vi "比率.vi"(10 "Fail 个数":dbl, 11 "Pass 个数":dbl) -> (1 "result":T1, 2 "fail 率":dbl, 3 "pass率":dbl)   [LabVIEW 2017]
panel:
  out "x/y 2":dbl
  out "x*y":dbl
  out "x/y":dbl
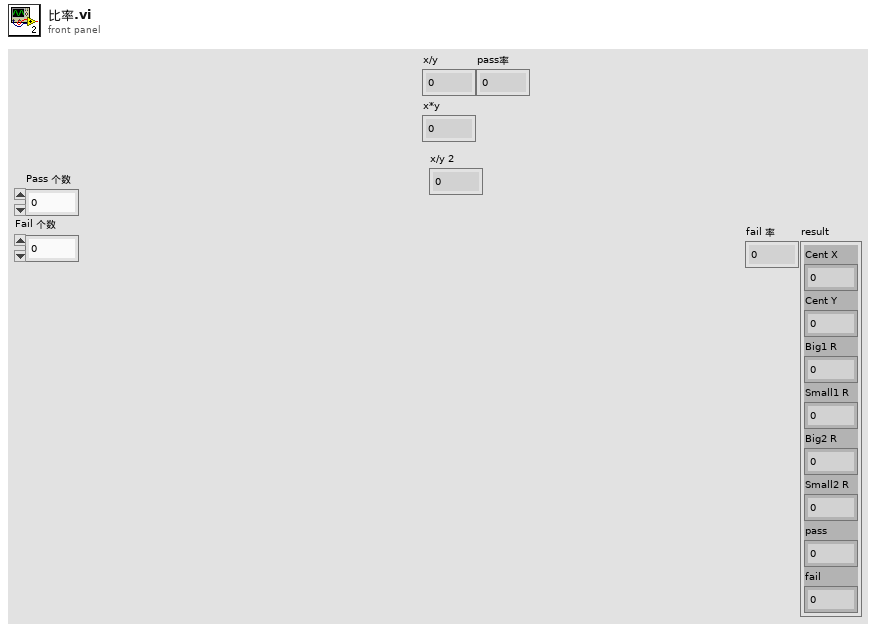
[diagram p1: front panel]
types:
  T1 = cluster{"Cent X":dbl, "Cent Y":dbl, "Big1 R":dbl, "Small1 R":dbl, "Big2 R":dbl, "Small2 R":dbl, "pass":dbl, "fail":dbl}
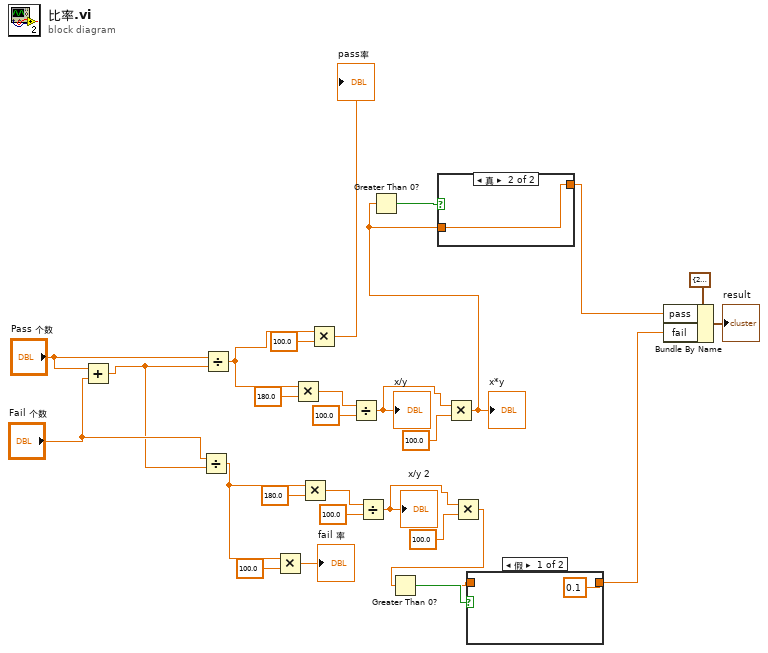
[diagram p0: block diagram]
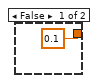
[diagram p3: hidden frame]
diagram:
  n1 = Add(x="Pass 个数", y="Fail 个数") -> (x+y=w19:dbl)
  n2 = Divide(x="Fail 个数", y=w19) -> (x/y=w10:dbl)
  n3 = Divide(x="Pass 个数", y=w19) -> (x/y=w13:dbl)
  n4 = Multiply(x=w10, y=100.0) -> (x*y=→"fail 率":dbl)
  n5 = Multiply(x=w13, y=180.0) -> (x*y=w23:dbl)
  n6 = Multiply(x=w10, y=180.0) -> (x*y=w16:dbl)
  n7 = Multiply(x=w13, y=100.0) -> (x*y=→"pass率":dbl)
  n8 = Divide(x=w23, y=100.0) -> (x/y=w22:dbl)
  "x/y" <- w22
  n9 = Divide(x=w16, y=100.0) -> (x/y=w17:dbl)
  "x/y 2" <- w17
  n10 = Multiply(x=w22, y=100.0) -> (x*y=w3:dbl)
  "x*y" <- w3
  n11 = Greater Than 0?(x=w3) -> (x > 0?=w9:bool)
  n12 = case shown="真" w9 {
    tunnel: [0.1 w29] -> w6
    tunnel: w3 -> [_ w29]
    frame False {
    }
    frame True {
    }
  }
  n13 = Multiply(x=w17, y=100.0) -> (x*y=w5:dbl)
  n14 = Greater Than 0?(x=w5) -> (x > 0?=w8:bool)
  n15 = case shown="假" w8 {
    tunnel: w5 -> [_ w31]
    tunnel: [0.1 w31] -> w4
    frame False {
    }
    frame True {
    }
  }
  n16 = Bundle By Name(cluster=T1 {"Cent X"=273.0, "Cent Y"=255.0, "Big1 R"=250.0, "Small1 R"=170.0, "Big2 R"=150.0, "Small2 R"=70.0, "pass"=0.1, "fail"=0.1} ("中心位置"), "pass"=w6, "fail"=w4) -> (→"result":T1)
